vi "SpecAn Noise Source Type Set.vi"(0 "VISA In":refnum<visa-resource-name>, 5 "Error In":errorcluster, 6 "Type":i32(ring) items=["Normal", "SNS"]) -> (14 "VISA Out":refnum<visa-resource-name>, 19 "Error Out":errorcluster)   [LabVIEW 2015]
uses:
  Controls/FGV Action SpecAn Model.ctl
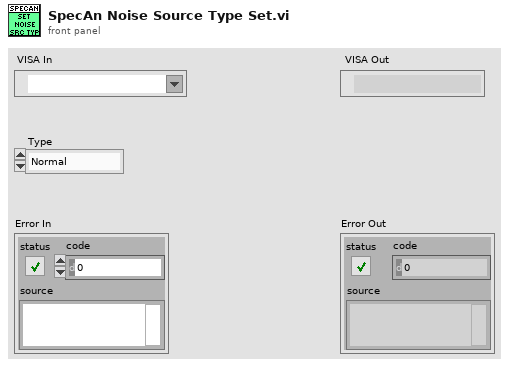
[diagram p1: front panel]
types:
  T1 = typedef "FGV Action SpecAn Model.ctl" = enum16{"Get", "Set"}
  T2 = typedef "SpecAn Model.ctl" = enum16{"E4440", "N9030"}
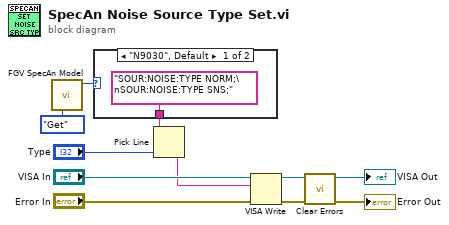
[diagram p0: block diagram]
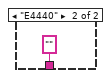
[diagram p2: hidden frame]
diagram:
  n1 = call "FGV SpecAn Model.vi"("Action"=FGV_Action_SpecAn_Model."Get") -> ("SA Model"=w2:T2)  [unwired: 6 in, 1 out]
  n2 = case shown="\"N9030\", Default" w2 {
    tunnel: ["SOUR:NOISE:TYPE NORM;\nSOUR:NOISE:TYPE SNS;" ("write buffer") "" ("write buffer")] -> w5
    frame "N9030", Default {
    }
    frame "E4440" {
    }
  }
  n3 = Pick Line(multi-line string=w5, line index="Type") -> (output string=w4:string)  [unwired: 1 in]
  n4 = VISA Write(VISA resource name="VISA In", write buffer=w4, error in (no error)="Error In") -> (VISA resource name out=→"VISA Out":refnum<visa-resource-name>, error out=w9:errorcluster)  [unwired: 1 out]
  n5 = call <vilib>:"Clear Errors.vi"("error in (no error)"=w9) -> ("error out"=→"Error Out":errorcluster)  [unwired: 5 in, 1 out]
